vi "Test Panel.vi"(8 "Error in":errorcluster, 9 "TDMS Name Mapping":T5={"FGEN Channel Mapping"=[["0", "Chn0"]], "DAQ Channel Mapping"=[["port0/line0", "Chn0"], ["port0/line1", "Chn1"], ["port0/line2", "Chn2"]], "FGEN Wfm List"=[["Wfm1", "FGEN_Wfm1"], ["Wfm2", "FGEN_Wfm2"]], "DAQ Wfm List"=[["Wfm1", "DAQ_Wfm1"], ["Wfm2", "DAQ_Wfm2"]]}, 10 "Wavefom Sequence":T4={"FGEN Wfm Sequence"=["Wfm1"], "DAQ Wfm Sequence"=["Wfm1"], "Loops"=[1]}, 11 "Resource Settings":T3={"FGEN Resource"="", "DAQmx Resource"="", "TDMS File Path"=path "", "Scope Resource"="", "Scope Config File Path"=path "", "Reference Position"=50.0, "Duration"=-1.0} {"Duration" format="%#_6ps"; "Reference Position" format="%#_g%"}) -> (0 "Error out":errorcluster, 2 "Plot Names":string[](array[string]), 3 "Captured Waveforms":T1(graph))   [LabVIEW 2025]
uses:
  Typedef/TDMS Name Mapping.ctl
  Typedef/Resource Settings.ctl
panel:
  in  "Stop":bool
  in  "Tab Control":T2(tab)
  # "FGEN - Scope - Digital DAQ Test Panel"
  # "Right-click the graph to export waveforms to file"
  # "* Negative duration will keep the original waveform length in the scope settings"
  # "* Make sure the number of elements in each array are match"
  # "This Test Panel can control FGEN and DAQ to generate a sequence of analog and \ndigital waveforms from a TDMS file. While generating, it can also control SCOPE to \ncapture multiple records according to the number of steps in the Waveform \nSequence (FGEN or DAQ).\n\nYou can choose to disable FGEN, DAQ or SCOPE function by leaving thier Resource \nNames blank. \n\nIf FGEN and DAQ are enabled, DAQ will arm the FGEN start trigger before it starts \ngeneration through the PXI backplane (implicit triggering). If only DAQ enabled,\nDAQ will start generation immediately.\n\nBefore start, prepare a TMDS waveform file that matches the TDMS Name Mapping:\n  - For FGEN:\n      - Refer to the FGEN Channel Mapping and FGEN Wfm List.\n      - FGEN will run with the Arbitrary Sequence mode and Single Trigger mode to \n         generate the waveforms in the FGEN Wfm Sequence. \n      - If want to enebale a marker event in the generated waveform, create custom  \n         properties on the TDMS group called \"Marker0\" and specify the marker0 position.\n         And make sure the \"Export Marker0 From File\" on this Test Panel is checked.\n      - If \"Export Marker0 From File\" is checked but no Marker0 properties in the FGEN\n         waveform TDMS group, it will not throw error but just disable the Marker0 event \n         for this waveform. \n      - Data will resampled to the highest sample rate among all the FGEN waveforms.\n  - For DAQ:\n     - Refer to the DAQ Channel Mapping and DAQ Wfm List\n     - The waveforms specified in the DAQ Wfm Sequence will be cascaded as one \n        waveform for each channel. \n     - Data will resampled to the highest sample rate among all the DAQ waveforms.\n\nThen, configure the FGEN and DAQ Sequence accordingly. Number of records to be \ncaptured by SCOPE will follow the number of steps in FGEN Waveform Sequence\nif FGEN is enabled. Otherwise, it follows the number of steps in the DAQ Waveform\nSequence.\n\nUse the InstrumentStudio to configure the settings of SCOPE first, and export the \nsettings as .niscopeconfig file. Then, you can use the file to configure the settings\nin this Test Panel."
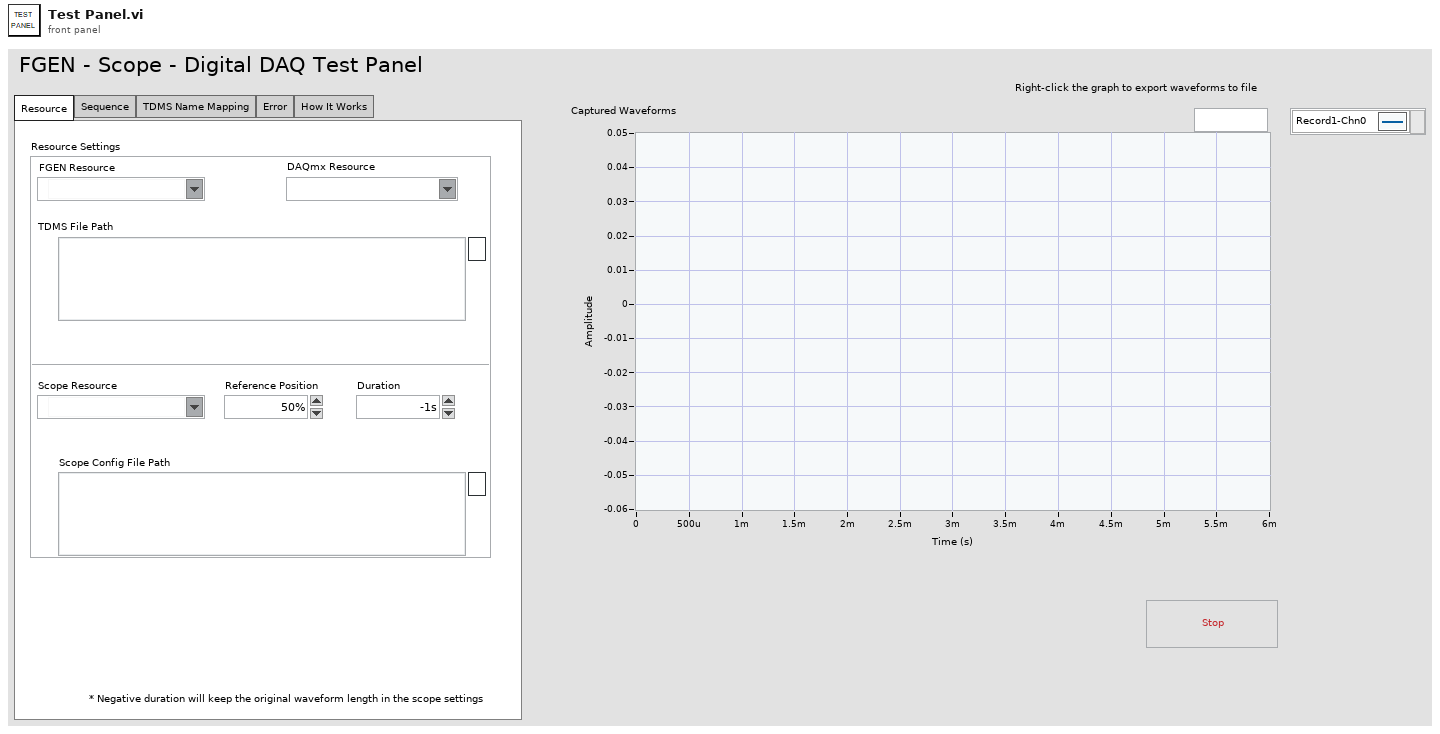
[diagram p1: front panel]
types:
  T1 = cluster{"relativeInitialX":dbl, "xIncrement":dbl, "wfm":dbl[]}[]
  T2 = enum32{"Resource", "Sequence", "TDMS Name Mapping", "Error", "How It Works"}
  T3 = typedef "Resource Settings.ctl" = cluster{"FGEN Resource":refnum<k15>, "DAQmx Resource":tag, "TDMS File Path":path, "Scope Resource":refnum<k15>, "Scope Config File Path":path, "Reference Position":dbl, "Duration":dbl}
  T4 = cluster{"FGEN Wfm Sequence":string[], "DAQ Wfm Sequence":string[], "Loops":i32[]}
  T5 = typedef "TDMS Name Mapping.ctl" = cluster{"FGEN Channel Mapping":string[][], "DAQ Channel Mapping":string[][], "FGEN Wfm List":string[][], "DAQ Wfm List":string[][]}
  T6 = typedef "Test Panel State Data.ctl" = cluster{"FGEN Resource":refnum<k15>, "DAQmx Tasks Session":cluster{"DO Task":refnum<k21>, "Ctr0 Task":refnum<k21>}, "Scope Resource":refnum<k15>, "FGEN Enabled?":bool, "DAQ Enabled?":bool, "Scope Enabled?":bool, "Max Total FGEN Wfm Duration (s)":dbl, "Number of Records":i32, "FGEN-DAQ Routing":cluster{"FGEN Start Trigger":string, "DAQ Trig Line":string}}
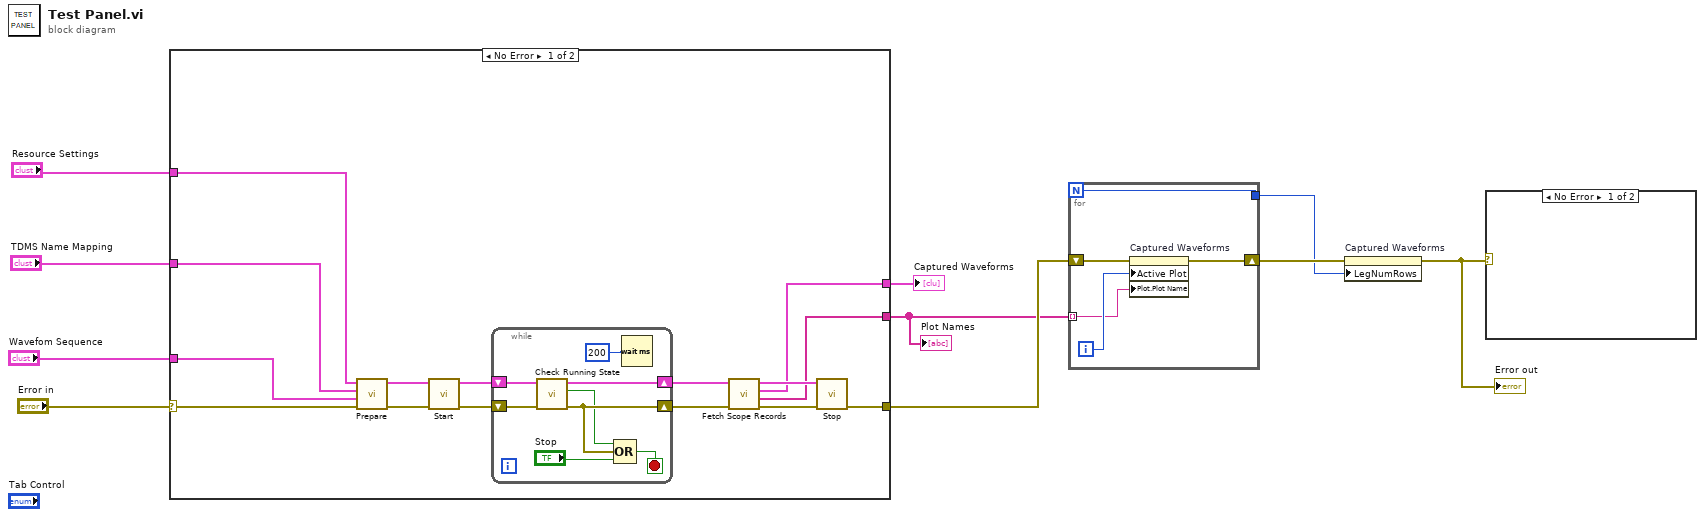
[diagram p0: block diagram]
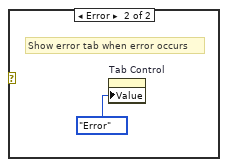
[diagram p3: hidden frame]
diagram:
  n1 = case shown="No Error" "Error in" {
    selector: "Error in" -> [w22 w34]
    tunnel: [w14 w34] -> w5
    tunnel: "Resource Settings" -> [w25 _]
    tunnel: "TDMS Name Mapping" -> [w24 _]
    tunnel: "Wavefom Sequence" -> [w23 _]
    tunnel: [w12 _] -> w7
    tunnel: [w11 _] -> w4
    frame No Error {
      n2 = call "Prepare.vi"("error in (no error)"=w22, "Wavefom Sequence"=w23, "TDMS Name Mapping"=w24, "Resource Settings"=w25) -> ("error out"=w21:errorcluster, "Panel State Data Out"=w19:T6)  [unwired: 6 in]
      n3 = call "Start.vi"("error in (no error)"=w21, "Panel State Data In"=w19) -> ("error out"=w20:errorcluster, "Panel State Data Out"=w17:T6)  [unwired: 7 in, 1 out]
      n4 = while {
        shift-right: [w30] -> w18
        shift-left: w20 -> [w33]
        shift-right: [w29] -> w15
        shift-left: w17 -> [w32]
        stop <- w31 stop-if-true
        n5 = call "Check Running State.vi"("error in (no error)"=w33, "Panel State Data In"=w32) -> ("error out"=w30:errorcluster, "Is Done?"=w27:bool, "Panel State Data Out"=w29:T6)  [unwired: 7 in]
        n6 = Compound Arithmetic op=OR(w27, w30, "Stop") -> (w31:bool)
        n7 = Wait (ms)(milliseconds to wait=u32 200) -> ()  [unwired: 1 out]
      }
      n8 = call "Fetch Scope Records.vi"("error in (no error)"=w18, "Panel State Data In"=w15) -> ("error out"=w16:errorcluster, "Plot Names"=w11:string[], "Captured Waveforms"=w12:T1, "Panel State Data Out"=w13:T6)  [unwired: 6 in]
      n9 = call "Stop.vi"("error in (no error)"=w16, "Panel State Data In"=w13) -> ("error out"=w14:errorcluster)  [unwired: 8 in, 1 out]
    }
    frame Error {
    }
  }
  "Captured Waveforms" <- w7
  "Plot Names" <- w4
  n10 = for {
    N -> [w35]
    tunnel: w4 -> [w37] mode=indexing
    shift-right: [w36] -> w3
    shift-left: w5 -> [w39]
    tunnel: [w35] -> w2
    i -> [w38]
    n11 = property on="Captured Waveforms" class="WFGraph (strict)"(error in=w39, "Active Plot"=w38, "Plot.Plot Name"=w37) -> (error out=w36:errorcluster)  [unwired: 1 in, 1 out]
  }
  n12 = property on="Captured Waveforms" class="WFGraph (strict)"(error in=w3, "LegNumRows"=w2) -> (error out=w1:errorcluster)  [unwired: 1 in, 1 out]
  "Error out" <- w1
  n13 = case shown="No Error" w1 {
    frame No Error {
    }
    frame Error {
      # "Show error tab when error occurs"
      n14 = property on="Tab Control" class="TabCtl (strict)"("Value"=T2."Error" ("Tab Control")) -> ()  [unwired: 2 in, 2 out]
    }
  }
